vi "build_DI_task.vi"(8 "error in":errorcluster) -> (0 "error out":errorcluster, 3 "task out":refnum<k21>)   [LabVIEW 2013]
uses:
  <vilib>/DAQmx/create/channels.llb/DAQmx Create Channel (DI-Digital Input).vi
  <resource>/objmgr/daqmx.rc
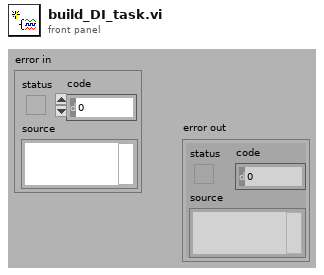
[diagram p1: front panel]
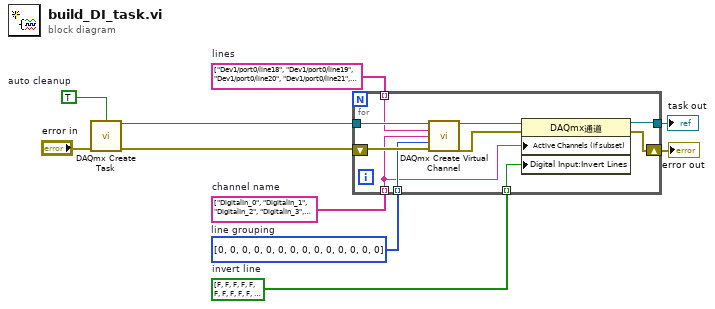
[diagram p0: block diagram]
diagram:
  w6 = bool[] [FALSE, FALSE, FALSE, FALSE, FALSE, FALSE, FALSE, FALSE, FALSE, FALSE, FALSE, FALSE, FALSE, FALSE]  # invert line
  w5 = i32[] [0, 0, 0, 0, 0, 0, 0, 0, 0, 0, 0, 0, 0, 0] items=["one channel for each line", "one channel for all lines"]  # line grouping
  w4 = string[] ["DigitalIn_0", "DigitalIn_1", "DigitalIn_2", "DigitalIn_3", "DigitalIn_4", "DigitalIn_5", "DigitalIn_6", "DigitalIn_7", "DigitalIn_8", "DigitalIn_9", "DigitalIn_10", "DigitalIn_11", "DigitalIn_12", "DigitalIn_13"]  # channel name
  w3 = string[] ["Dev1/port0/line18", "Dev1/port0/line19", "Dev1/port0/line20", "Dev1/port0/line21", "Dev1/port0/line22", "Dev1/port0/line23", "Dev1/port0/line24", "Dev1/port0/line25", "Dev1/port0/line26", "Dev1/port0/line27", "Dev1/port0/line28", "Dev1/port0/line29", "Dev1/port0/line30", "Dev1/port0/line31"]  # lines
  w8 = TRUE  # auto cleanup
  n1 = call <vilib>:"DAQmx Create Task.vi"("auto cleanup"=w8, "error in"="error in") -> ("task out"=w7:refnum<k21>, "error out"=w9:errorcluster)  [unwired: 12 in]
  n2 = for {
    tunnel: w7 -> [w20]
    tunnel: w6 -> [w14] mode=indexing
    tunnel: w5 -> [w17] mode=indexing
    tunnel: w4 -> [w13] mode=indexing
    tunnel: w3 -> [w18] mode=indexing
    tunnel: [w15] -> w2
    shift-right: [w11] -> w1
    shift-left: w9 -> [w19]
    n3 = call-poly <vilib>:"DAQmx Create Virtual Channel.vi"("task in"=w20, "lines"=w18, "name to assign"=w13, "line grouping"=w17, "error in"=w19) -> ("task out"=w16:refnum<k21>, "error out"=w12:errorcluster)  [unwired: 9 in]
    n4 = property class="DAQmx通道"(reference=w16, error in=w12, "Active Channels (if subset)"=w13, "Digital Input:Invert Lines"=w14) -> (reference out=w15:refnum<k21>, error out=w11:errorcluster)
  }
  "error out" <- w1
  "task out" <- w2
